vi "Get Path to Base Test VI.vi"() -> (3 "Path":path)   [LabVIEW 2020]
doc: "Returns path to Base Test VI. Do not change the location of this helper."
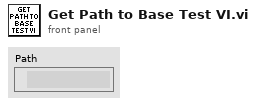
[diagram p1: front panel]
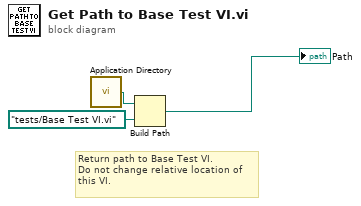
[diagram p0: block diagram]
diagram:
  # "Return path to Base Test VI.\nDo not change relative location of\nthis VI."
  n1 = call <vilib>:"Application Directory.vi"() -> ("Application Directory"=w1:path)
  n2 = Build Path(base path=w1, name or relative path=path "tests/Base Test VI.vi") -> (appended path=→"Path":path)
